vi "CONFIG NEO ARM ACTUATORS.vi"(8 "error in (no error)":errorcluster, 10 "MotorControlDevRef":T2, 11 "RefName":string) -> (0 "error out":errorcluster={"status"=TRUE, "code"=-1, "source"="Motor Controller Configure All Settings Enhanced: 1 or more configs failed"}, 3 "MotorControlDeviceRef out":T2={"DeviceStatus"={"status"=FALSE, "code"=0, "source"=""}, "Type"=enum."PWM", "PWM"={"PWM Channel"=enum."Invalid", "DeadBand"={"Name"="", "maxPositivePwm"=0, "minPositivePwm"=0, "centerPwm"=0, "maxNegativePwm"=0, "minNegativePwm"=0, "angularRange"=0}}, "CAN"={"Device Number"=0, "SetOutput VI Ref"=variant, "GetOutput VI Ref"=variant, "Enable VI Ref"=variant, "Disable VI Ref"=variant, "Data"=variant}, "Invert"=FALSE, "DIO PWM"={"PWM \"Enable\" Channel"=enum."Invalid", "DIOChannel"=enum."Invalid", "PWM Rate"=0.0}})   [LabVIEW 2020]
uses:
  <vilib>/Rock Robotics/WPI/MotorControl/WPI_MotorControlDeviceRef.ctl
  <vilib>/Rock Robotics/WPI/MotorControl/WPI_MotorControlType.ctl
  <vilib>/Rock Robotics/SystemInterfaces/DIO/FPGA_DIOPWMChannel.ctl
  <vilib>/Rock Robotics/WPI/PWM/WPI_PWMDeadband.ctl
  <vilib>/Rock Robotics/SystemInterfaces/DIO/FPGA_DIOChannel.ctl
  <vilib>/Rock Robotics/WPI/ThirdParty/REV Robotics/REVLib/Typedef/Spark MAX Idle Mode.ctl
  <vilib>/Rock Robotics/WPI/ThirdParty/REV Robotics/REVLib/Typedef/Spark MAX Motor Type.ctl
  <vilib>/Rock Robotics/WPI/ThirdParty/REV Robotics/REVLib/Typedef/Spark MAX Limit Direction.ctl
  <vilib>/Rock Robotics/WPI/ThirdParty/REV Robotics/REVLib/Typedef/Spark MAX Limit Switch Polarity.ctl
  Robot Global Data.vi
panel:
  in  "Idle Mode":T1=enum."Brake"
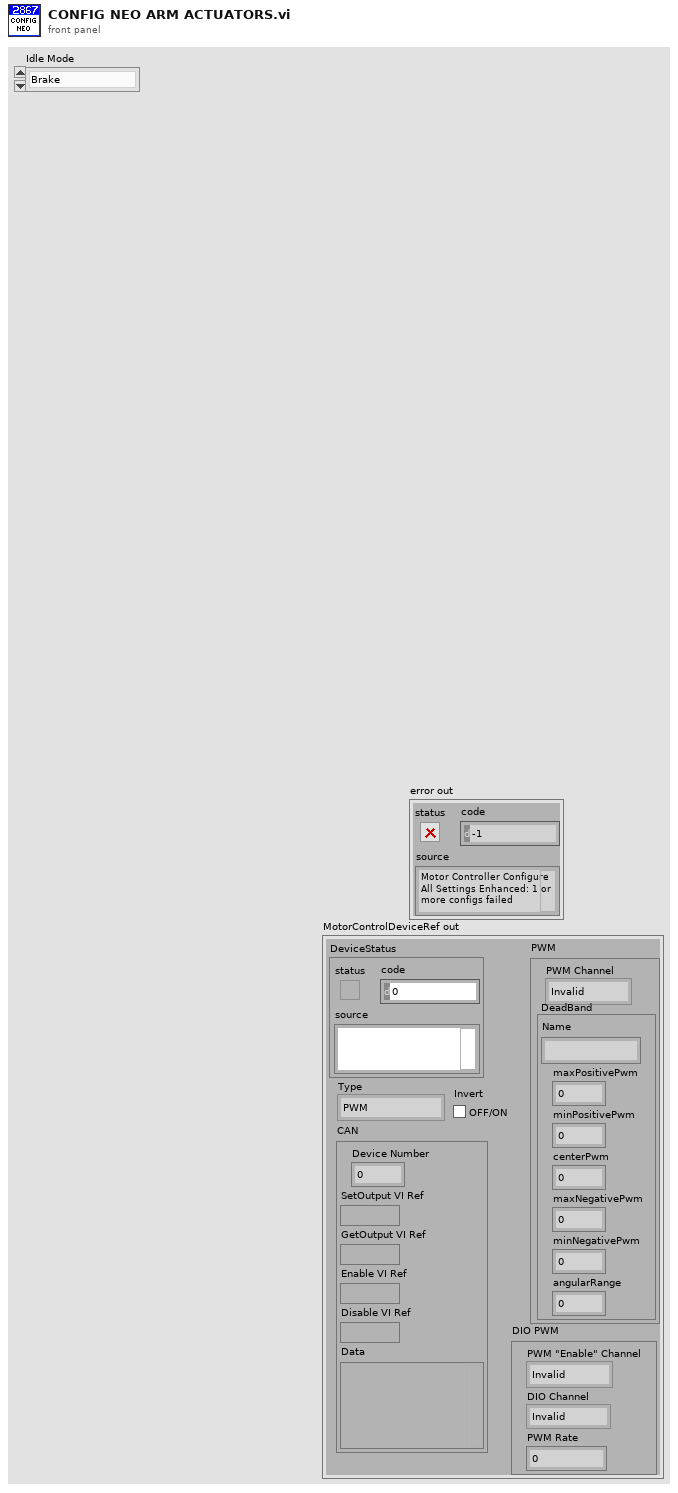
[diagram p1: front panel]
types:
  T1 = typedef "Spark MAX Idle Mode.ctl" = enum16{"Coast", "Brake"}
  T2 = typedef "WPI_MotorControlDeviceRef.ctl" = cluster{"DeviceStatus":errorcluster, "Type":T3, "PWM":cluster{"PWM Channel":T4, "DeadBand":T5}, "CAN":cluster{"Device Number":u8, "SetOutput VI Ref":variant, "GetOutput VI Ref":variant, "Enable VI Ref":variant, "Disable VI Ref":variant, "Data":variant}, "Invert":bool, "DIO PWM":cluster{"PWM \"Enable\" Channel":T4, "DIOChannel":T6, "PWM Rate":dbl}}
  T3 = typedef "WPI_MotorControlType.ctl" = enum16{"PWM", "CAN", "DIO PWM"}
  T4 = typedef "FPGA_DIOPWMChannel.ctl" = enum8{"PWM 0", "PWM 1", "PWM 2", "PWM 3", "PWM 4", "PWM 5", "PWM 6", "PWM 7", "PWM 8", "PWM 9", "PWM MXP 0", "PWM MXP 1", "PWM MXP 2", "PWM MXP 3", "PWM MXP 4", "PWM MXP 5", "PWM MXP 6", "PWM MXP 7", "PWM MXP 8", "PWM MXP 9", "Invalid"}
  T5 = typedef "WPI_PWMDeadband.ctl" = cluster{"Name":string, "maxPositivePwm":i32, "minPositivePwm":i32, "centerPwm":i32, "maxNegativePwm":i32, "minNegativePwm":i32, "angularRange":u16}
  T6 = typedef "FPGA_DIOChannel.ctl" = enum8{"DIO 0", "DIO 1", "DIO 2", "DIO 3", "DIO 4", "DIO 5", "DIO 6", "DIO 7", "DIO 8", "DIO 9", "DIO MXP 0", "DIO MXP 1", "DIO MXP 2", "DIO MXP 3", "DIO MXP 4", "DIO MXP 5", "DIO MXP 6", "DIO MXP 7", "DIO MXP 8", "DIO MXP 9", "DIO MXP 10", "DIO MXP 11", "DIO MXP 12", "DIO MXP 13", "DIO MXP 14", "DIO MXP 15", "SPI Port CS1", "SPI Port CS2", "SPI Port CS3", "SPI Port MISO", "SPI Port MOSI", "Invalid"}
  T7 = cluster{"MIN":dbl, "MAX":dbl, "convert arm inches to revs":dbl}
  T8 = typedef "Spark MAX Limit Switch Polarity.ctl" = enum16{"Normally Open", "Normally Closed"}
  T9 = typedef "Spark MAX Motor Type.ctl" = enum16{"Brushed", "Brushless"}
  T10 = typedef "Spark MAX Limit Direction.ctl" = enum16{"Forward Limit", "Reverse Limit"}
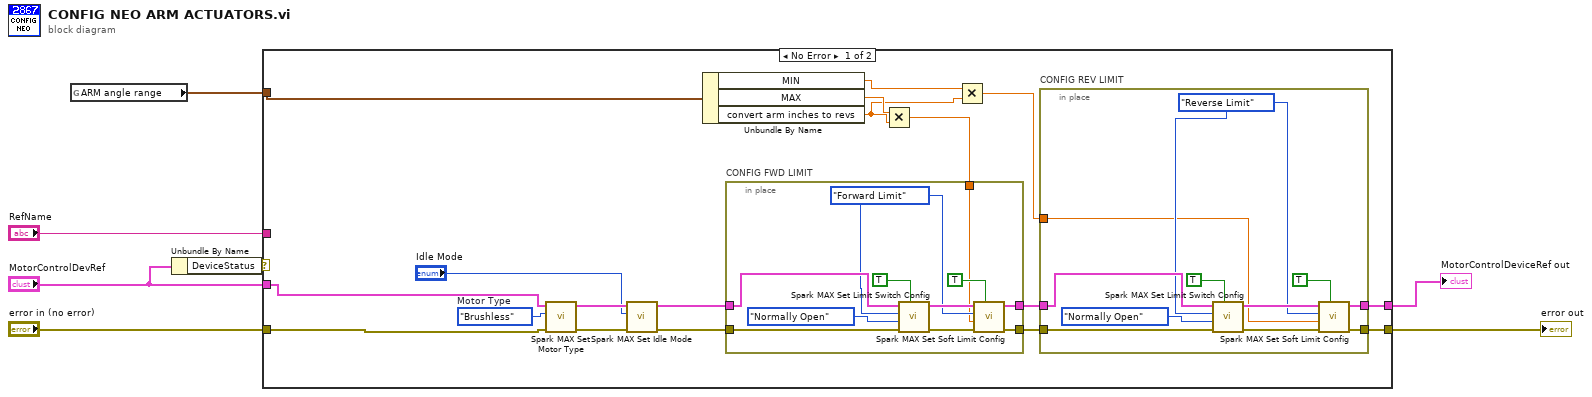
[diagram p0: block diagram]
diagram:
  n1 = global read "Robot Global Data.vi" "ARM angle range"() -> (w1:T7)
  n2 = Unbundle By Name("MotorControlDevRef") -> ("DeviceStatus"=w4:errorcluster)
  n3 = case shown="No Error" w4 {
    tunnel: [w25 _] -> w7
    tunnel: "RefName" -> [_ _]
    tunnel: "MotorControlDevRef" -> [w16 _]
    tunnel: [w15 _] -> w3
    tunnel: "error in (no error)" -> [w8 _]
    tunnel: w1 -> [w14 _]
    frame No Error {
      w19 = Spark_MAX_Motor_Type."Brushless"  # Motor Type
      n4 = call <vilib>:"Spark MAX Set Motor Type.vi"("error in (no error)"=w8, "Motor Type"=w19, "MotorControlDevRef"=w16) -> ("error out"=w22:errorcluster, "MotorControlDeviceRef"=w24:T2)  [unwired: 7 in]
      n5 = call <vilib>:"Spark MAX Set Idle Mode.vi"("error in (no error)"=w22, "Idle Mode"="Idle Mode", "MotorControlDeviceRef in"=w24) -> ("error out"=w21:errorcluster, "MotorControlDeviceRef out"=w23:T2)  [unwired: 7 in]
      n6 = Unbundle By Name(w14) -> ("MIN"=w9:dbl, "MAX"=w12:dbl, "convert arm inches to revs"=w10:dbl)
      n7 = Multiply(x=w12, y=w10) -> (x*y=w13:dbl)
      n8 = in-place "CONFIG FWD LIMIT" {
        in-place-border: w23 -> [w47]
        in-place-border: w21 -> [w46]
        in-place-border: [w44] -> w18
        in-place-border: [w42] -> w17
        in-place-border: w13 -> [w37]
        w38 = Spark_MAX_Limit_Direction."Forward Limit" ("Soft Limit Switch")
        n9 = call <vilib>:"Spark MAX Set Limit Switch Config.vi"("Enabled? (T)"=TRUE, "error in (no error)"=w46, "Polarity (Normally Open)"=Spark_MAX_Limit_Switch_Polarity."Normally Open", "Limit Switch"=w38, "MotorControlDeviceRef in"=w47) -> ("error out"=w43:errorcluster, "MotorControlDeviceRef out"=w45:T2)  [unwired: 5 in]
        n10 = call <vilib>:"Spark MAX Set Soft Limit Config.vi"("Enabled? (T)"=TRUE, "error in (no error)"=w43, "Soft Limit (0)"=w37, "Soft Limit Switch"=w38, "MotorControlDeviceRef in"=w45) -> ("error out"=w42:errorcluster, "MotorControlDeviceRef out"=w44:T2)  [unwired: 5 in]
      }
      n11 = Multiply(x=w9, y=w10) -> (x*y=w11:dbl)
      n12 = in-place "CONFIG REV LIMIT" {
        in-place-border: [w32] -> w25
        in-place-border: w18 -> [w36]
        in-place-border: w17 -> [w35]
        in-place-border: [w33] -> w15
        in-place-border: w11 -> [w26]
        w27 = Spark_MAX_Limit_Direction."Reverse Limit" ("Soft Limit Switch")
        n13 = call <vilib>:"Spark MAX Set Limit Switch Config.vi"("Enabled? (T)"=TRUE, "error in (no error)"=w35, "Polarity (Normally Open)"=Spark_MAX_Limit_Switch_Polarity."Normally Open", "Limit Switch"=w27, "MotorControlDeviceRef in"=w36) -> ("error out"=w31:errorcluster, "MotorControlDeviceRef out"=w34:T2)  [unwired: 5 in]
        n14 = call <vilib>:"Spark MAX Set Soft Limit Config.vi"("Enabled? (T)"=TRUE, "error in (no error)"=w31, "Soft Limit (0)"=w26, "Soft Limit Switch"=w27, "MotorControlDeviceRef in"=w34) -> ("error out"=w32:errorcluster, "MotorControlDeviceRef out"=w33:T2)  [unwired: 5 in]
      }
    }
    frame Error {
    }
  }
  "error out" <- w7
  "MotorControlDeviceRef out" <- w3
